vi "_CSMOFGV Obtain.vi"(7 "Allowed Messages(Empty for all)":string[](array[string]), 8 "Error in":errorcluster caption="Error in (no error)", 11 "Name(\"\" to use uuid) in":string) -> (0 "Error out":errorcluster, 1 "Create(T)/Cached(F)":bool, 3 "CSM-Obj":T1={"Requested Name"="", "Module Name"="", "Mode"=enum."Stand Alone", "Queue"=refnum, "CSM-Data"=refnum, "User Event"=refnum, "Status Change Event"=refnum, "Allowed Messages"=[], "Mode-Data"=refnum, "Group Name"="", "Exit Event"=refnum}, 4 "Name":string)   [LabVIEW 2020, in "Communicable State Machine.lvlib"]
uses:
  Communicable State Machine.lvlib
  _CSMObj.ctl
  Priority Queue.lvclass
  _CSM_MODE.ctl
  _CSMObj-Data.ctl
  _CSM Status Change Event Data.ctl
  _CSMObj-ModeData.ctl
  Priority Queue.lvclass/Priority Queue.ctl
  _CSMOFGVOPER.ctl
  global-CSMQ FGV Change Flag.vi
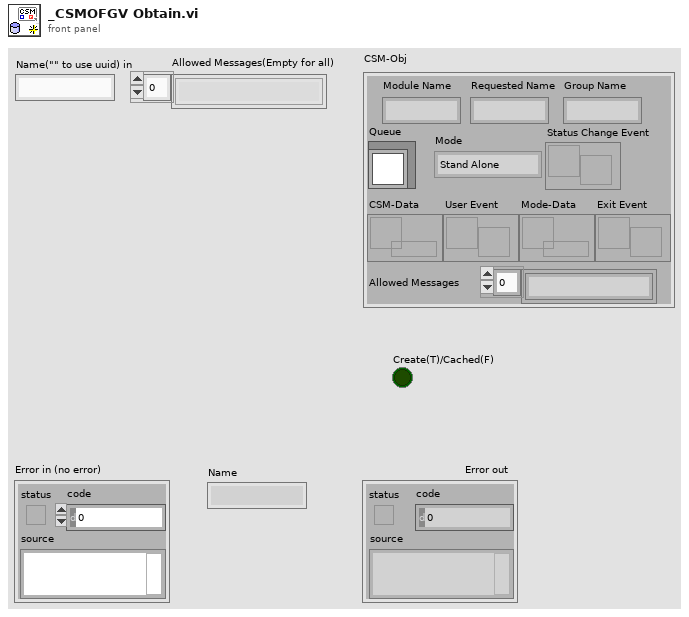
[diagram p1: front panel]
types:
  T1 = typedef "Communicable State Machine.lvlib/_CSMObj.ctl" = cluster{"Requested Name":string, "Module Name":string, "Mode":T2, "Queue":refnum<class "Priority Queue.lvclass">, "CSM-Data":refnum<data-value>, "User Event":refnum<user-event>, "Status Change Event":refnum<user-event>, "Allowed Messages":string[], "Mode-Data":refnum<data-value>, "Group Name":string, "Exit Event":refnum<user-event>}
  T2 = typedef "Communicable State Machine.lvlib/_CSM_MODE.ctl" = enum16{"Not Exist", "Stand Alone", "CSM", "Worker Agent", "Worker", "Chain", "Chain Node"}
  T3 = typedef "Communicable State Machine.lvlib/_CSMOFGVOPER.ctl" = enum16{"Create If not Exist", "Get By Name", "List", "Check If Name Exists", "Release", "Module Status", "Create Status Event Handler", "Destroy Status Event Handler"}
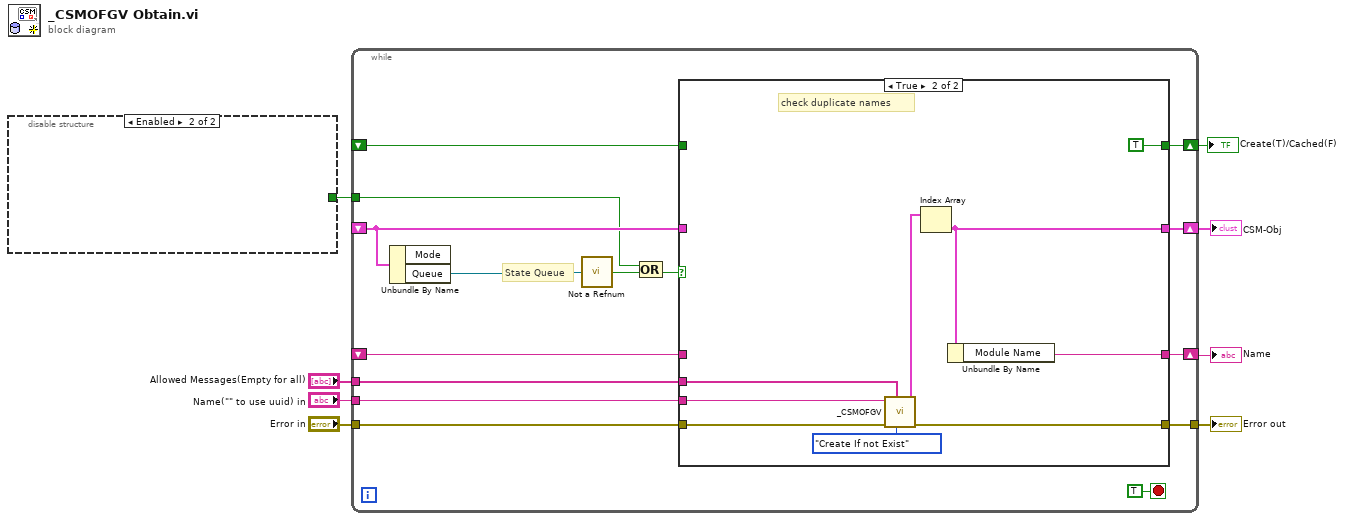
[diagram p0: block diagram]
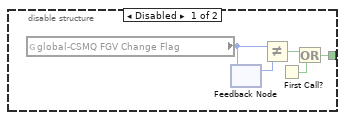
[diagram p2: hidden frame]
diagram:
  n1 = disable-structure shown="Enabled" {
    disable-tunnel: [w13 _] -> w4
    frame Disabled {
      n2 = global read "global-CSMQ FGV Change Flag.vi" "global-CSMQ FGV Change Flag"() -> (w9:u64)
      n3 = feedback #1() -> (w10:u64)  [unwired: 1 in]
      n4 = feedback-in #1(w9) -> ()
      n5 = Not Equal?(x=w9, y=w10) -> (x != y?=w12:bool)
      n6 = First Call?() -> (First Call?: T/F=w11:bool)
      n7 = Or(x=w12, y=w11) -> (x .or. y?=w13:bool)
    }
    frame Enabled {
    }
  }
  n8 = while {
    shift-right: [w26] -> w5
    shift-left: _ -> [w21]
    tunnel: "Error in" -> [w25]
    tunnel: [w24] -> w7
    tunnel: "Name(\"\" to use uuid) in" -> [w22]
    shift-right: [w19] -> w1
    shift-left: _ -> [w18]
    tunnel: w4 -> [w17]
    shift-right: [w15] -> w3
    shift-left: _ -> [w16]
    tunnel: "Allowed Messages(Empty for all)" -> [w14]
    stop <- TRUE stop-if-true
    # "State Queue"
    n9 = Unbundle By Name(w21) -> ("Queue"=w20:refnum<class "Priority Queue.lvclass">)  [unwired: 1 out]
    n10 = call "Not a Refnum.vi"("Priority Queue.lvclass"=w20) -> ("NaN/Path/Refnum?"=w27:bool)  [unwired: 4 in]
    n11 = Compound Arithmetic op=OR(w17, w27) -> (w23:bool)
    n12 = case shown="True" w23 {
      tunnel: [w31 w34] -> w26
      tunnel: w21 -> [w31 _]
      tunnel: w25 -> [w30 w36]
      tunnel: [w30 w38] -> w24
      tunnel: w22 -> [_ w32]
      tunnel: [w29 w33] -> w19
      tunnel: w18 -> [w29 _]
      tunnel: w16 -> [_ _]
      tunnel: [_ TRUE] -> w15
      tunnel: w14 -> [_ w35]
      frame False {
      }
      frame True {
        # "check duplicate names"
        n13 = call "_CSMOFGV.vi"("Operation"=_CSMOFGVOPER."Create If not Exist", "Allowed Messages(Empty for all)"=w35, "Error in"=w36, "Name(\"\" to use uuid) in"=w32) -> ("Error out"=w38:errorcluster, "Array"=w40:T1[])  [unwired: 5 in, 1 out]
        n14 = Index Array(array=w40) -> (element=w34:T1)  [unwired: 1 in]
        n15 = Unbundle By Name(w34) -> ("Module Name"=w33:string)
      }
    }
  }
  "Error out" <- w7
  "CSM-Obj" <- w5
  "Name" <- w1
  "Create(T)/Cached(F)" <- w3
